vi "Periodic Tasks.vi"(8 "error in":errorcluster) -> ()   [LabVIEW 2014]
doc: "This VI runs in parallel to other tasks. It can contain as many user-defined periodic loops as you need. These can carry out PID or other sorts of timed response."
uses:
  <vilib>/Platform/TimedLoop/XDataNode/timing_clust.ctl
  <vilib>/Platform/TimedLoop/XDataNode/nitl_modes.ctl
  <vilib>/Platform/TimedLoop/XDataNode/wakeup.ctl
  <vilib>/Rock Robotics/WPI/SafetyOutput/WPI_SafetyOutputConfigMenu.ctl
  <vilib>/platform/TimedLoop/XDataNode/XDataNode.xnode
  <vilib>/Platform/TimedLoop/XDataNode/XDNodeRunTimeDep.lvlib
  <vilib>/functionblocks/FB Core/FB Core.xnode
  <vilib>/functionblocks/Edge Detection/One Shot Rising with Input/One Shot Rising with Input.vi
  <vilib>/functionblocks/NI_FunctionBlock Libraries.lvlib
panel:
  out "Lift_Motors":cluster{"Lift_Motor1":dbl, "Lift_Motor2":dbl}(graph)={"Lift_Motor1"=-0.065, "Lift_Motor2"=-0.05376856590023428}
  out "Lift_Motor_Output":dbl=-0.05376856590023428
  in  "Lift_2_(Rear)_Open_Loop":bool
  in  "Lift 2 (Rear) Control Inputs":T1={"Kp"=0.004, "Ki"=0.0, "i upper"=0.3, "i lower"=-0.3, "Output upper"=1.0, "Output lower"=-0.2} {"Kp" step=0.0005}
  in  "Lower_Position_Limit":dbl
  in  "Upper_Position_Limit":dbl=5000.0
  out "Lift_1_Open_Loop":bool
  out "Lift_1_Terms":T2={"Feedforward Term"=0.0, "P Term "=-0.065, "I Term"=0.0}
  in  "Min_Lift_Threshold":dbl=0.1 format="%#_13g"
  out "Lift 2(Rear)":cluster{"Target":dbl, "Feedback":dbl}(graph)={"Target"=-0.4421414750585697, "Feedback"=13.0}
  out "Lift 1(Front)":cluster{"Target":dbl, "Feedback":dbl}(graph)={"Target"=0.0, "Feedback"=13.0}
  in  "Common_Control_Inputs":T1={"Kp"=0.0009, "Ki"=0.0, "i upper"=0.3, "i lower"=-0.3, "Output upper"=1.0, "Output lower"=-1.0}
  in  "Rear_Right_Control":cluster{"kP":dbl, "kI":dbl}={"kP"=0.0009, "kI"=0.0001}
  in  "Rear_Left_Control":cluster{"kP":dbl, "kI":dbl}={"kP"=0.0009, "kI"=0.0001}
  in  "Front_Right_Control":cluster{"kP":dbl, "kI":dbl}={"kP"=0.0009, "kI"=0.0001}
  in  "Front_Left_Control":cluster{"kP":dbl, "kI":dbl}={"kP"=0.0009, "kI"=0.0001}
  out "Rear_Right":cluster{"Target":dbl, "Feedback":dbl}(graph)
  out "Rear_Left":cluster{"Target":dbl, "Feedback":dbl}(graph)
  out "Front_Right":cluster{"Target":dbl, "Feedback":dbl}(graph)={"Target"=-0.0, "Feedback"=0.0}
  out "Wheel Output":T3(graph)={"Encoder Velocity"=-0.060933706792958474, -0.07682162051881043, "Encoder Velocity"=-0.12463025207176147, "Encoder Velocity"=-0.06995107080703702}
  out "Rear_Right_Terms":T2={"Feedforward Term"=0.0, "P Term "=0.0, "I Term"=-0.06995107080703702}
  out "Rear_Left_Terms":T2={"Feedforward Term"=0.0, "P Term "=0.0, "I Term"=-0.12463025207176147}
  out "Front_Right_Terms":T2={"Feedforward Term"=0.0, "P Term "=-0.0, "I Term"=-0.07682162051881043}
  out "Front_Left_Terms":T2={"Feedforward Term"=0.0, "P Term "=0.0, "I Term"=-0.060933706792958474}
  in  "Lift 1 (Front) Control Inputs":T1={"Kp"=0.005, "Ki"=0.0, "i upper"=0.3, "i lower"=-0.3, "Output upper"=1.0, "Output lower"=-1.0}
  in  "Open Loop Max Speed":dbl=1.0
  in  "Motor Effort Axis":dbl[](array[numeric])=[0.0, 0.0, 0.0, 0.0, 0.0] format="%_6g"
  in  "Speed Axis":dbl[](array[numeric])=[-2000.0, -300.0, 0.0, 300.0, 200.0] format="%_6g"
  out "Rear_Right_Error":dbl
  out "Rear_Left_Error":dbl
  out "Front_Right_Error":dbl=-0.0
  out "Front_Left_Error":dbl
  out "Front_Left":cluster{"Target":dbl, "Feedback":dbl}(graph)
  out "YawRate":dbl(graph)=-0.06208816528320313
  out "Angle":dbl(graph)=-0.0012461343125000001
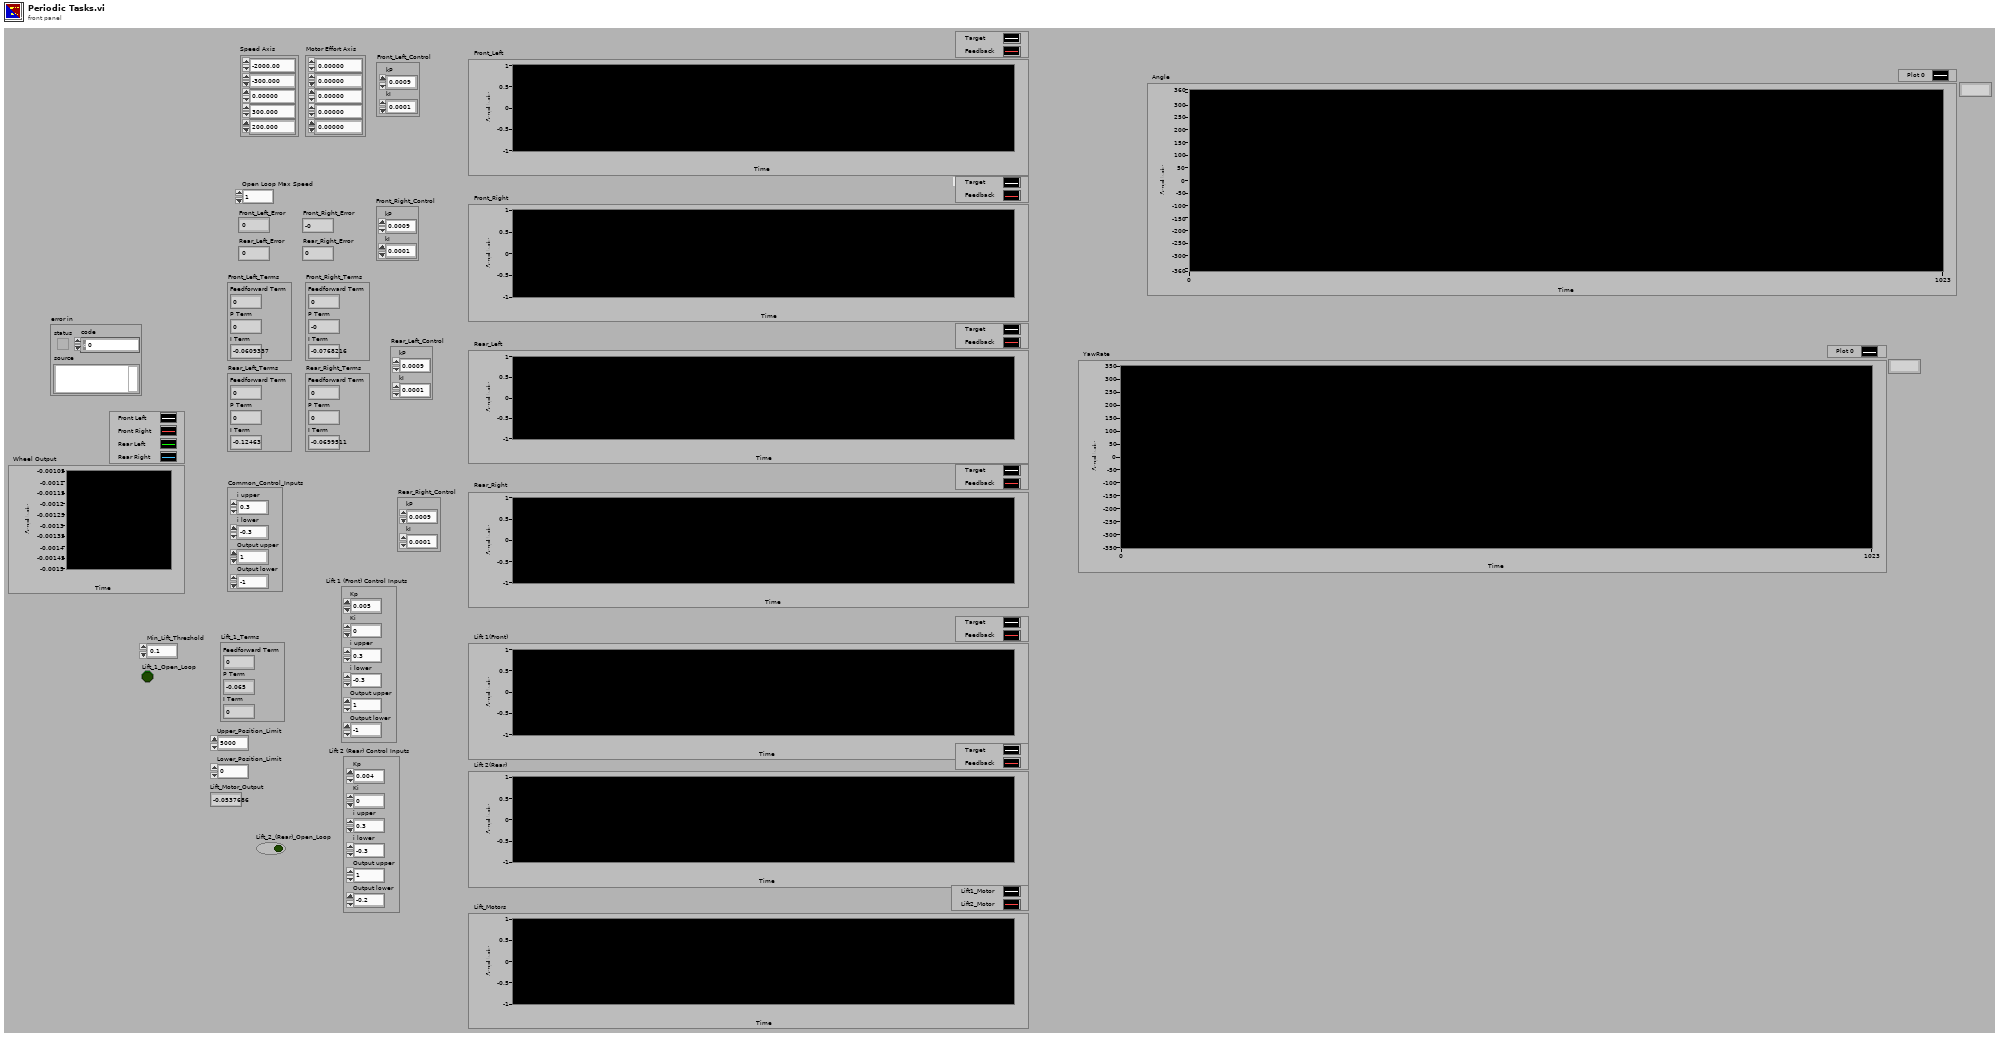
[diagram p1: front panel]
types:
  T1 = cluster{"Kp":dbl, "Ki":dbl, "i upper":dbl, "i lower":dbl, "Output upper":dbl, "Output lower":dbl}
  T2 = cluster{"Feedforward Term":dbl, "P Term ":dbl, "I Term":dbl}
  T3 = cluster{"Encoder Velocity":dbl, dbl, "Encoder Velocity":dbl, "Encoder Velocity":dbl}
  T4 = typedef "XDNodeRunTimeDep.lvlib/timing_clust.ctl" = cluster{"Expected End [f-1]":u64, "Actual End [f-1]":u64, "Finished Late? [f-1]":bool, "Expected End [i-1]":u64, "Actual End [i-1]":u64, "Finished Late? [i-1]":bool, "Expected Start [i]":u64, "Actual Start [i]":u64, "Expected Start [f]":u64, "Actual Start [f]":u64, "Source Name":string, "Structure Name":string, "Period":i64, "Deadline":i64, "Offset":i64, "Start":i64, "Priority":i32, "Timeout":i32, "Mode":T5, "Wakeup Reason":T6, "Error":errorcluster, "Source Type":string, "Secondary Source Type":string, "Global End Time":u64, "Global Start Time":u64, "Frame Duration":u64, "Iteration Duration":u64, "Assigned CPU":i32, "I/O Scan Engine Mode":u32}
  T5 = typedef "XDNodeRunTimeDep.lvlib/nitl_modes.ctl" = enum32{"No Change", "Process missed periods, maintain original phase", "Discard missed periods, maintain original phase", "Process missed periods, ignore original phase", "Discard missed periods, ignore original phase"}
  T6 = typedef "XDNodeRunTimeDep.lvlib/wakeup.ctl" = enum32{"Normal", "Aborted", "Asynchronous wakeup", "Timing source error", "Timed loop error", "Timeout"}
  T7 = cluster{"Front Left Target":dbl, "Front Right Target":dbl, "Rear Left Target":dbl, "Rear Right Target":dbl}
  T8 = typedef "WPI_SafetyOutputConfigMenu.ctl" = enum16{"Enable", "Disable"}
  T9 = cluster{"Front Left":dbl, "Front Right":dbl, "Rear Left":dbl, "Rear Right":dbl}
  T10 = typedef "WPI_GyroDevRef.ctl" = cluster{"DevStatus":errorcluster, "Analog Module":T11, "Analog Channel":T12, "Offset":dbl, "Gain (VoltsPerDegree/Second)":dbl}
  T11 = typedef "FPGA_TypedefAnalogModule.ctl" = enum16{"Controller 1"}
  T12 = typedef "FPGA_AIChannel.ctl" = enum8{"AI 0", "AI 1", "AI 2", "AI 3", "AI MXP 0", "AI MXP 1", "AI MXP 2", "AI MXP 3", "Invalid"}
  T13 = typedef "WPI_EncoderDevRef.ctl" = cluster{"DevStatus":errorcluster, "EncoderIndex":T14, "CounterIndex":T15, "DistancePerCount":dbl, "Decoding Type":T16}
  T14 = typedef "FPGA_EncoderIdx.ctl" = enum8{"Enc 0", "Enc 1", "Enc 2", "Enc 3", "Enc 4", "Enc 5", "Enc 6", "Enc 7", "Invalid"}
  T15 = typedef "FPGA_CounterCtrSystemIndex.ctl" = enum8{"Ctr 0", "Ctr 1", "Ctr 2", "Ctr 3", "Ctr 4", "Ctr 5", "Ctr 6", "Ctr 7", "Invalid"}
  T16 = typedef "WPI_EncoderType.ctl" = enum16{"1x", "2x", "4x"}
  T17 = typedef "WPI_MotorControlDeviceRef.ctl" = cluster{"DeviceStatus":errorcluster, "Type":T18, "PWM":cluster{"Controller":T19, "PWM Channel":T20, "DeadBand":T21}, "CAN":cluster{"Device Number":u8, "Control Mode":T22, "Semaphore":T23, "Max Vout":dbl, "TalonSRX Control Mode":T24}, "Invert":bool, "TransformRef":T25, "InvTransformRef":T25}
  T18 = typedef "WPI_MotorControlType.ctl" = enum16{"PWM", "CAN", "CANTalonSRX"}
  T19 = typedef "FPGA_TypedefDigitalModule.ctl" = enum16{"Controller 1"}
  T20 = typedef "FPGA_DIOPWMChannel.ctl" = enum8{"PWM 0", "PWM 1", "PWM 2", "PWM 3", "PWM 4", "PWM 5", "PWM 6", "PWM 7", "PWM 8", "PWM 9", "PWM MXP 0", "PWM MXP 1", "PWM MXP 2", "PWM MXP 3", "PWM MXP 4", "PWM MXP 5", "PWM MXP 6", "PWM MXP 7", "PWM MXP 8", "PWM MXP 9", "Invalid"}
  T21 = typedef "WPI_PWMDeadband.ctl" = cluster{"Name":string, "maxPositivePwm":i32, "minPositivePwm":i32, "centerPwm":i32, "maxNegativePwm":i32, "minNegativePwm":i32, "angularRange":u16}
  T22 = typedef "WPI_CANJaguar_ControlMode.ctl" = enum8{"Percent VBus", "Current", "Speed", "Position", "Voltage"}
  T23 = typedef "Semaphore RefNum" = refnum<k1>
  T24 = typedef "WPI_CANTalonSRX_APIControlMode.ctl" = enum8{"Percent VBus", "Speed", "Position", "Slave", "Unchanged / Invalid"}
  T25 = typedef "WPI_PWMTransform_ConPane.ctl" = refnum<vi>
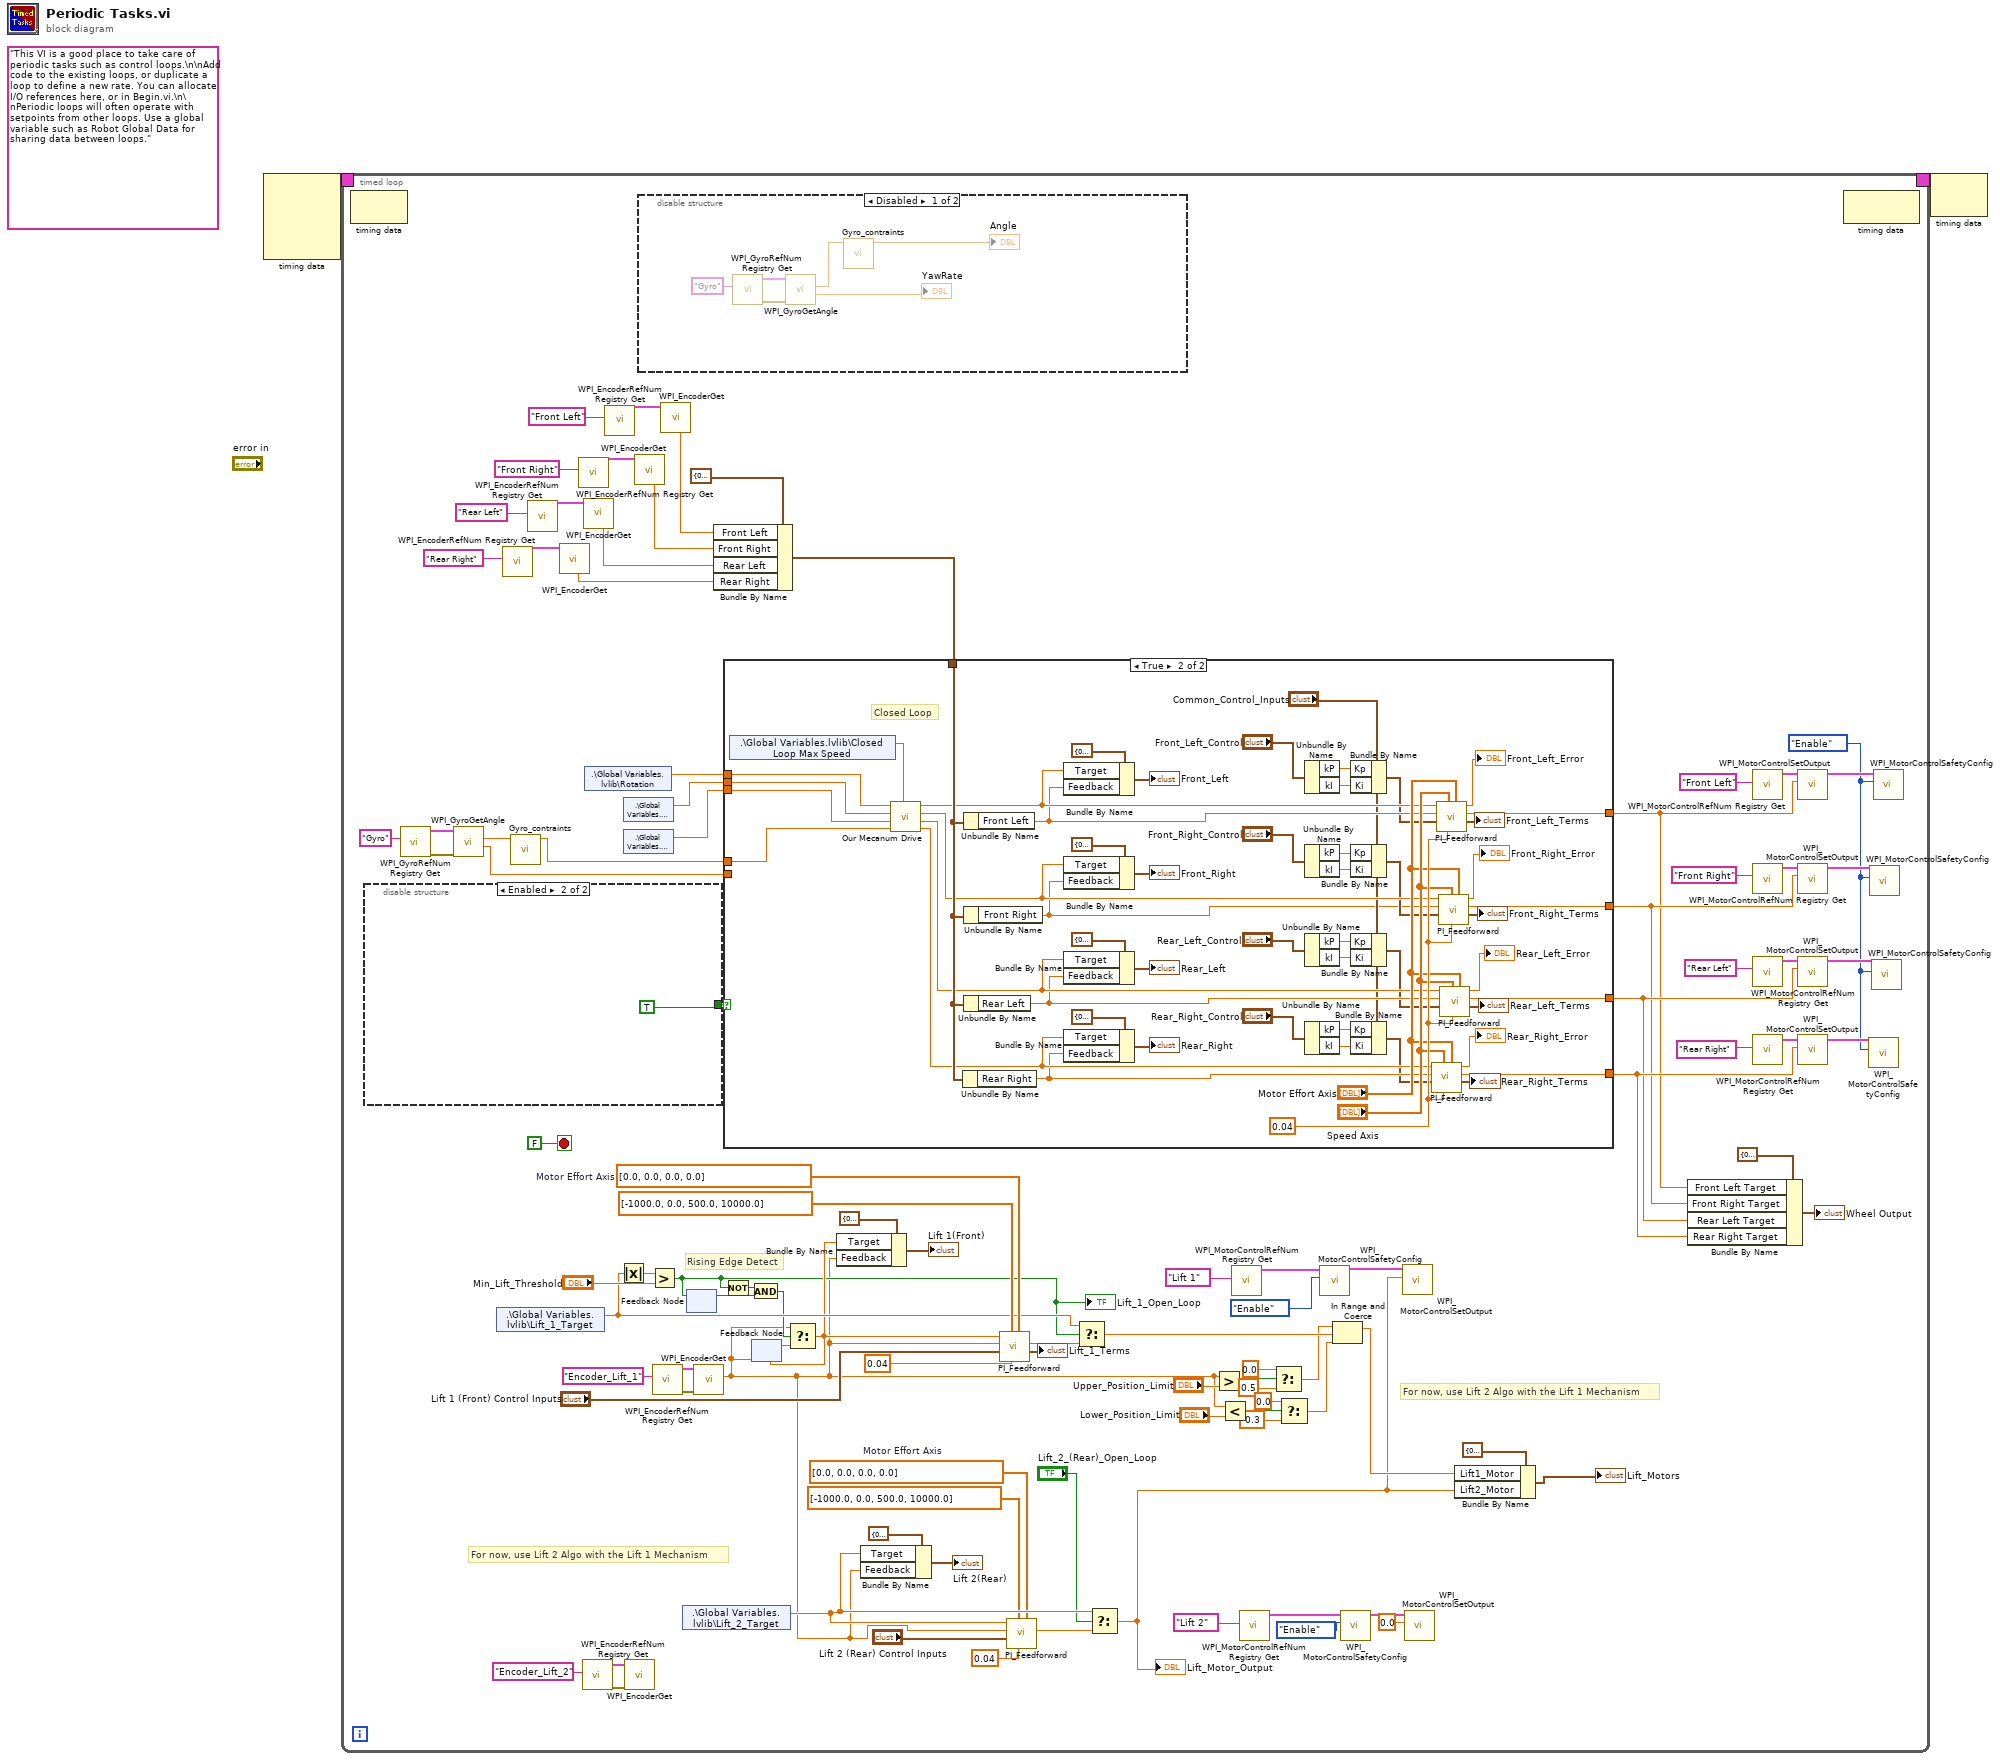
[diagram p0: block diagram]
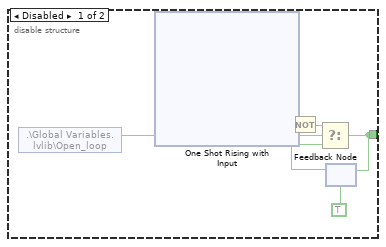
[diagram p2: hidden frame]
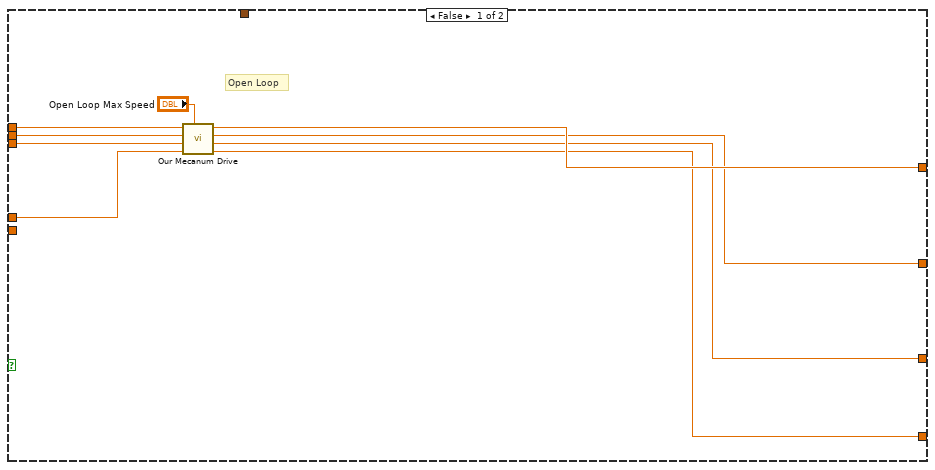
[diagram p3: hidden frame]
diagram:
  (unwired) "This VI is a good place to take care of periodic tasks such as control loops.\n\nAdd code to the existing loops, or duplicate a loop to define a new rate. You can allocate I/O references here, or in Begin.vi.\n\nPeriodic loops will often operate with setpoints from other loops. Use a global variable such as Robot Global Data for sharing data between loops."
  n1 = node-c288() -> (w2:T4)  [unwired: 4 in]
  n2 = timed-loop {
    timing: w2 -> [_]
    timing-out: [_] -> w1
    stop <- FALSE stop-if-true
    w8 = dbl[] [0.0, 0.0, 0.0, 0.0]  # Motor Effort Axis
    w53 = dbl[] [0.0, 0.0, 0.0, 0.0]  # Motor Effort Axis
    w88 = WPI_SafetyOutputConfigMenu."Enable" ("mode")
    # "For now, use Lift 2 Algo with the Lift 1 Mechanism"
    # "For now, use Lift 2 Algo with the Lift 1 Mechanism"
    # "Rising Edge Detect"
    n3 = node-c288() -> ()  [unwired: 1 in, 1 out]
    n4 = disable-structure shown="Enabled" {
      disable-tunnel: [w105 TRUE] -> w67
      frame Disabled {
        n5 = shared-variable ".\\Global Variables.lvlib\\Open_loop"() -> (w109:bool)  [unwired: 1 in, 1 out]
        n6 = xnode "One Shot Rising with Input"("input"=w109) -> ("output"=w108:bool)  [unwired: 1 in, 1 out]
        n7 = feedback #1(TRUE) -> (w106:bool)
        n8 = Not(x=w106) -> (.not. x?=w107:bool)
        n9 = Select(t=w107, s=w108, f=w106) -> (s? t:f=w105:bool)
        n10 = feedback-in #1(w105) -> ()
      }
      frame Enabled {
      }
    }
    n11 = call <vilib>:"WPI_GyroRefNum Registry Get.vi"("refnum name"="Gyro") -> ("error out"=w66:errorcluster, "GyroDevRef"=w65:T10)  [unwired: 9 in]
    n12 = call <vilib>:"WPI_GyroGetAngle.vi"("error in (no error)"=w66, "GyroDevRef"=w65) -> ("Angular Rate"=w61:dbl, "Angle"=w63:dbl)  [unwired: 6 in, 2 out]
    n13 = shared-variable ".\\Global Variables.lvlib\\Lift_1_Target"() -> (w35:dbl)  [unwired: 1 in, 1 out]
    n14 = call <vilib>:"WPI_EncoderRefNum Registry Get.vi"("refnum name"="Rear Right") -> ("EncoderDevRef"=w71:T13)  [unwired: 9 in, 1 out]
    n15 = call "Gyro_contraints.vi"("angle"=w63) -> ("final angle"=w62:dbl)  [unwired: 10 in]
    n16 = call <vilib>:"WPI_EncoderRefNum Registry Get.vi"("refnum name"="Rear Left") -> ("EncoderDevRef"=w68:T13)  [unwired: 9 in, 1 out]
    n17 = call <vilib>:"WPI_EncoderGet.vi"("EncoderDevRef"=w71) -> ("Rate"=w47:dbl)  [unwired: 5 in, 5 out]
    n18 = call <vilib>:"WPI_EncoderRefNum Registry Get.vi"("refnum name"="Front Right") -> ("EncoderDevRef"=w72:T13)  [unwired: 9 in, 1 out]
    n19 = call <vilib>:"WPI_EncoderRefNum Registry Get.vi"("refnum name"="Encoder_Lift_2") -> ("error out"=w56:errorcluster, "EncoderDevRef"=w57:T13)  [unwired: 9 in]
    n20 = call <vilib>:"WPI_EncoderGet.vi"("EncoderDevRef"=w68) -> ("Rate"=w46:dbl)  [unwired: 5 in, 5 out]
    n21 = shared-variable ".\\Global Variables.lvlib\\Rotation"() -> (w87:dbl)  [unwired: 1 in, 1 out]
    n22 = call <vilib>:"WPI_EncoderRefNum Registry Get.vi"("refnum name"="Front Left") -> ("EncoderDevRef"=w76:T13)  [unwired: 9 in, 1 out]
    n23 = Absolute Value(x=w35) -> (abs(x)=w39:dbl)
    n24 = shared-variable ".\\Global Variables.lvlib\\Y"() -> (w86:dbl)  [unwired: 1 in, 1 out]
    n25 = shared-variable ".\\Global Variables.lvlib\\X"() -> (w85:dbl)  [unwired: 1 in, 1 out]
    n26 = call <vilib>:"WPI_EncoderGet.vi"("error in (no error)"=w56, "EncoderDevRef"=w57) -> ()  [unwired: 4 in, 6 out]
    n27 = call <vilib>:"WPI_EncoderGet.vi"("EncoderDevRef"=w72) -> ("Rate"=w45:dbl)  [unwired: 5 in, 5 out]
    n28 = disable-structure shown="Disabled" {
      frame Disabled {
        n29 = call <vilib>:"WPI_GyroRefNum Registry Get.vi"("refnum name"="Gyro") -> ("error out"=w217:errorcluster, "GyroDevRef"=w216:T10)  [unwired: 9 in]
        n30 = call <vilib>:"WPI_GyroGetAngle.vi"("error in (no error)"=w217, "GyroDevRef"=w216) -> ("Angular Rate"=→"YawRate":dbl, "Angle"=w213:dbl)  [unwired: 6 in, 2 out]
        n31 = call "Gyro_contraints.vi"("angle"=w213) -> ("final angle"=→"Angle":dbl)  [unwired: 10 in]
      }
      frame Enabled {
      }
    }
    n32 = Greater?(x=w39, y="Min_Lift_Threshold") -> (0:w17:bool)
    "Lift_1_Open_Loop" <- w17
    n33 = call <vilib>:"WPI_EncoderRefNum Registry Get.vi"("refnum name"="Encoder_Lift_1") -> ("error out"=w59:errorcluster, "EncoderDevRef"=w58:T13)  [unwired: 9 in]
    n34 = call <vilib>:"WPI_EncoderGet.vi"("EncoderDevRef"=w76) -> ("Rate"=w75:dbl)  [unwired: 5 in, 5 out]
    n35 = shared-variable ".\\Global Variables.lvlib\\Lift_2_Target"() -> (w40:dbl)  [unwired: 1 in, 1 out]
    n36 = feedback-in #2(w17) -> ()
    n37 = feedback #2() -> (w36:bool)  [unwired: 1 in]
    n38 = call <vilib>:"WPI_EncoderGet.vi"("error in (no error)"=w59, "EncoderDevRef"=w58) -> ("Distance"=w10:dbl)  [unwired: 4 in, 5 out]
    n39 = Bundle By Name(cluster=T9 {"Front Left"=0.0, "Front Right"=-0.0, "Rear Left"=9.0, "Rear Right"=-0.0} ("Cluster"), "Front Left"=w75, "Front Right"=w45, "Rear Left"=w46, "Rear Right"=w47) -> (w89:T9)
    n40 = Not(x=w17) -> (.not. x?=w37:bool)
    n41 = case shown="True" w67 {
      tunnel: w89 -> [_ w210]
      tunnel: w87 -> [w156 w209]
      tunnel: w86 -> [w155 w208]
      tunnel: w85 -> [w154 w207]
      tunnel: [w153 w206] -> w3
      tunnel: [w152 w203] -> w4
      tunnel: [w151 w202] -> w5
      tunnel: [w150 w199] -> w6
      tunnel: w62 -> [w149 w195]
      tunnel: w61 -> [_ _]
      frame False {
        # "Open Loop"
        n42 = call "Our Mecanum Drive.vi"("Max Output"="Open Loop Max Speed", "Gyro Angle"=w149, "X"=w154, "Y"=w155, "Rotation"=w156) -> ("Rear Right"=w150:dbl, "Rear Left"=w151:dbl, "Front Right"=w152:dbl, "Front Left"=w153:dbl)  [unwired: 3 in]
      }
      frame True {
        w198 = 0.04 ("dT")
        # "Closed Loop"
        n43 = shared-variable ".\\Global Variables.lvlib\\Closed Loop Max Speed"() -> (w211:dbl)  [unwired: 1 in, 1 out]
        n44 = call "Our Mecanum Drive.vi"("Max Output"=w211, "Gyro Angle"=w195, "X"=w207, "Y"=w208, "Rotation"=w209) -> ("Rear Right"=w184:dbl, "Rear Left"=w182:dbl, "Front Right"=w180:dbl, "Front Left"=w189:dbl)  [unwired: 3 in]
        n45 = Unbundle By Name(w210) -> ("Rear Right"=w183:dbl)
        n46 = Unbundle By Name(w210) -> ("Front Left"=w188:dbl)
        n47 = Unbundle By Name(w210) -> ("Front Right"=w158:dbl)
        n48 = Unbundle By Name(w210) -> ("Rear Left"=w181:dbl)
        n49 = Bundle By Name(cluster=cluster{"Target":dbl, "Feedback":dbl} {"Target"=0.0, "Feedback"=0.0}, "Target"=w189, "Feedback"=w188) -> (→"Front_Left":cluster{"Target":dbl, "Feedback":dbl})
        n50 = Bundle By Name(cluster=cluster{"Target":dbl, "Feedback":dbl} {"Target"=0.0, "Feedback"=0.0}, "Target"=w180, "Feedback"=w158) -> (→"Front_Right":cluster{"Target":dbl, "Feedback":dbl})
        n51 = Bundle By Name(cluster=cluster{"Target":dbl, "Feedback":dbl} {"Target"=0.0, "Feedback"=0.0}, "Target"=w182, "Feedback"=w181) -> (→"Rear_Left":cluster{"Target":dbl, "Feedback":dbl})
        n52 = Bundle By Name(cluster=cluster{"Target":dbl, "Feedback":dbl} {"Target"=0.0, "Feedback"=0.0}, "Target"=w184, "Feedback"=w183) -> (→"Rear_Right":cluster{"Target":dbl, "Feedback":dbl})
        n53 = Unbundle By Name("Front_Left_Control") -> ("kP"=w169:dbl, "kI"=w168:dbl)
        n54 = Unbundle By Name("Front_Right_Control") -> ("kP"=w167:dbl, "kI"=w160:dbl)
        n55 = Unbundle By Name("Rear_Left_Control") -> ("kP"=w162:dbl, "kI"=w161:dbl)
        n56 = Unbundle By Name("Rear_Right_Control") -> ("kP"=w166:dbl, "kI"=w165:dbl)
        n57 = Bundle By Name(cluster="Common_Control_Inputs", "Kp"=w169, "Ki"=w168) -> (w171:T1)
        n58 = Bundle By Name(cluster="Common_Control_Inputs", "Kp"=w167, "Ki"=w160) -> (w172:T1)
        n59 = Bundle By Name(cluster="Common_Control_Inputs", "Kp"=w162, "Ki"=w161) -> (w173:T1)
        n60 = Bundle By Name(cluster="Common_Control_Inputs", "Kp"=w166, "Ki"=w165) -> (w174:T1)
        n61 = call "PI_Feedforward.vi"("Motor Effort Axis"="Motor Effort Axis", "dT"=w198, "Position Axis"="Speed Axis", "Control Inputs"=w174, "Feed Back"=w183, "Target"=w184) -> ("Term Indicators"=→"Rear_Right_Terms":T2, "Output"=w199:dbl, "Error"=→"Rear_Right_Error":dbl)  [unwired: 3 in]
        n62 = call "PI_Feedforward.vi"("Motor Effort Axis"="Motor Effort Axis", "dT"=w198, "Position Axis"="Speed Axis", "Control Inputs"=w171, "Feed Back"=w188, "Target"=w189) -> ("Term Indicators"=→"Front_Left_Terms":T2, "Output"=w206:dbl, "Error"=→"Front_Left_Error":dbl)  [unwired: 3 in]
        n63 = call "PI_Feedforward.vi"("Motor Effort Axis"="Motor Effort Axis", "dT"=w198, "Position Axis"="Speed Axis", "Control Inputs"=w172, "Feed Back"=w158, "Target"=w180) -> ("Term Indicators"=→"Front_Right_Terms":T2, "Output"=w203:dbl, "Error"=→"Front_Right_Error":dbl)  [unwired: 3 in]
        n64 = call "PI_Feedforward.vi"("Motor Effort Axis"="Motor Effort Axis", "dT"=w198, "Position Axis"="Speed Axis", "Control Inputs"=w173, "Feed Back"=w181, "Target"=w182) -> ("Term Indicators"=→"Rear_Left_Terms":T2, "Output"=w202:dbl, "Error"=→"Rear_Left_Error":dbl)  [unwired: 3 in]
      }
    }
    n65 = And(x=w37, y=w36) -> (x .and. y?=w34:bool)
    n66 = feedback #3(w10) -> (w33:dbl)
    n67 = Select(t=w10, s=w34, f=w33) -> (s? t:f=w32:dbl)
    n68 = feedback-in #3(w32) -> ()
    n69 = Bundle By Name(cluster=cluster{"Target":dbl, "Feedback":dbl} {"Target"=0.0, "Feedback"=0.0}, "Target"=w32, "Feedback"=w10) -> (→"Lift 1(Front)":cluster{"Target":dbl, "Feedback":dbl})
    n70 = Bundle By Name(cluster=cluster{"Target":dbl, "Feedback":dbl} {"Target"=0.0, "Feedback"=0.0}, "Target"=w40, "Feedback"=w10) -> (→"Lift 2(Rear)":cluster{"Target":dbl, "Feedback":dbl})
    n71 = call "PI_Feedforward.vi"("Motor Effort Axis"=w53, "dT"=0.04, "Position Axis"=dbl[] [-1000.0, 0.0, 500.0, 10000.0], "Control Inputs"="Lift 1 (Front) Control Inputs", "Feed Back"=w10, "Target"=w32) -> ("Term Indicators"=→"Lift_1_Terms":T2, "Output"=w49:dbl)  [unwired: 3 in, 1 out]
    n72 = call "PI_Feedforward.vi"("Motor Effort Axis"=w8, "dT"=0.04, "Position Axis"=dbl[] [-1000.0, 0.0, 500.0, 10000.0], "Control Inputs"="Lift 2 (Rear) Control Inputs", "Feed Back"=w10, "Target"=w40) -> ("Output"=w48:dbl)  [unwired: 3 in, 2 out]
    n73 = Select(t=w35, s=w17, f=w49) -> (s? t:f=w28:dbl)
    n74 = Select(t=w40, s="Lift_2_(Rear)_Open_Loop", f=w48) -> (s? t:f=w9:dbl)
    "Lift_Motor_Output" <- w9
    n75 = Greater?(x=w10, y="Upper_Position_Limit") -> (0:w24:bool)
    n76 = Less?(x=w10, y="Lower_Position_Limit") -> (x < y?=w25:bool)
    n77 = call <vilib>:"WPI_MotorControlRefNum Registry Get.vi"("refnum name"="Lift 1") -> ("MotorControlDevRef"=w83:T17)  [unwired: 9 in, 1 out]
    n78 = call <vilib>:"WPI_MotorControlRefNum Registry Get.vi"("refnum name"="Lift 2") -> ("MotorControlDevRef"=w80:T17)  [unwired: 9 in, 1 out]
    n79 = Select(t=0.0, s=w24, f=0.5) -> (s? t:f=w23:dbl)
    n80 = Select(t=0.0, s=w25, f=-0.3) -> (s? t:f=w20:dbl)
    n81 = call <vilib>:"WPI_MotorControlSafetyConfig.vi"("mode"=WPI_SafetyOutputConfigMenu."Enable", "MotorControlDevRef"=w83) -> ("MotorControlDevRef"=w82:T17)  [unwired: 8 in, 1 out]
    n82 = In Range and Coerce(upper limit=w23, x=w28, lower limit=w20) -> (coerced(x)=w12:dbl)  [unwired: 1 out]
    n83 = call <vilib>:"WPI_MotorControlSafetyConfig.vi"("mode"=WPI_SafetyOutputConfigMenu."Enable", "MotorControlDevRef"=w80) -> ("MotorControlDevRef"=w79:T17)  [unwired: 8 in, 1 out]
    n84 = call <vilib>:"WPI_MotorControlSetOutput.vi"("Output"=w9, "MotorControlDevRef"=w82) -> ()  [unwired: 7 in, 3 out]
    n85 = call <vilib>:"WPI_MotorControlSetOutput.vi"("Output"=0.0, "MotorControlDevRef"=w79) -> ()  [unwired: 7 in, 3 out]
    n86 = Bundle By Name(cluster=cluster{"Lift1_Motor":dbl, "Lift2_Motor":dbl} {"Lift1_Motor"=0.0, "Lift2_Motor"=0.0}, "Lift1_Motor"=w12, "Lift2_Motor"=w9) -> (→"Lift_Motors":cluster{"Lift1_Motor":dbl, "Lift2_Motor":dbl})
    n87 = Bundle By Name(cluster=T7 {"Front Left Target"=0.0, "Front Right Target"=0.0, "Rear Left Target"=0.0, "Rear Right Target"=0.0}, "Front Left Target"=w3, "Front Right Target"=w4, "Rear Left Target"=w5, "Rear Right Target"=w6) -> (→"Wheel Output":T7)
    n88 = call <vilib>:"WPI_MotorControlRefNum Registry Get.vi"("refnum name"="Front Left") -> ("MotorControlDevRef"=w98:T17)  [unwired: 9 in, 1 out]
    n89 = call <vilib>:"WPI_MotorControlRefNum Registry Get.vi"("refnum name"="Front Right") -> ("MotorControlDevRef"=w96:T17)  [unwired: 9 in, 1 out]
    n90 = call <vilib>:"WPI_MotorControlRefNum Registry Get.vi"("refnum name"="Rear Left") -> ("MotorControlDevRef"=w97:T17)  [unwired: 9 in, 1 out]
    n91 = call <vilib>:"WPI_MotorControlRefNum Registry Get.vi"("refnum name"="Rear Right") -> ("MotorControlDevRef"=w95:T17)  [unwired: 9 in, 1 out]
    n92 = call <vilib>:"WPI_MotorControlSetOutput.vi"("Output"=w3, "MotorControlDevRef"=w98) -> ("MotorControlDevRef"=w94:T17)  [unwired: 7 in, 2 out]
    n93 = call <vilib>:"WPI_MotorControlSetOutput.vi"("Output"=w4, "MotorControlDevRef"=w96) -> ("MotorControlDevRef"=w93:T17)  [unwired: 7 in, 2 out]
    n94 = call <vilib>:"WPI_MotorControlSetOutput.vi"("Output"=w5, "MotorControlDevRef"=w97) -> ("MotorControlDevRef"=w92:T17)  [unwired: 7 in, 2 out]
    n95 = call <vilib>:"WPI_MotorControlSetOutput.vi"("Output"=w6, "MotorControlDevRef"=w95) -> ("MotorControlDevRef"=w91:T17)  [unwired: 7 in, 2 out]
    n96 = node-c288() -> ()  [unwired: 1 in, 1 out]
    n97 = call <vilib>:"WPI_MotorControlSafetyConfig.vi"("mode"=w88, "MotorControlDevRef"=w91) -> ()  [unwired: 8 in, 2 out]
    n98 = call <vilib>:"WPI_MotorControlSafetyConfig.vi"("mode"=w88, "MotorControlDevRef"=w93) -> ()  [unwired: 8 in, 2 out]
    n99 = call <vilib>:"WPI_MotorControlSafetyConfig.vi"("mode"=w88, "MotorControlDevRef"=w92) -> ()  [unwired: 8 in, 2 out]
    n100 = call <vilib>:"WPI_MotorControlSafetyConfig.vi"("mode"=w88, "MotorControlDevRef"=w94) -> ()  [unwired: 8 in, 2 out]
  }
  n101 = node-c288(w1) -> ()  [unwired: 1 out]
